vi "GetLastCharacterInformation.vi"(8 "error in (no error)":errorcluster, 10 "Right Text Information":T1, 11 "EAN-13 In":refnum<class "EAN-13.lvclass">) -> (0 "error out":errorcluster, 2 "Text Information":T1, 3 "EAN-13 out":refnum<class "EAN-13.lvclass">)   [LabVIEW 2013, in "BarCodes.lvlib" / "EAN-13.lvclass"]
uses:
  EAN-13.lvclass
  BarCode/TextPosition.ctl
  BarCodes.lvlib
  BarCode/BarCode.lvclass
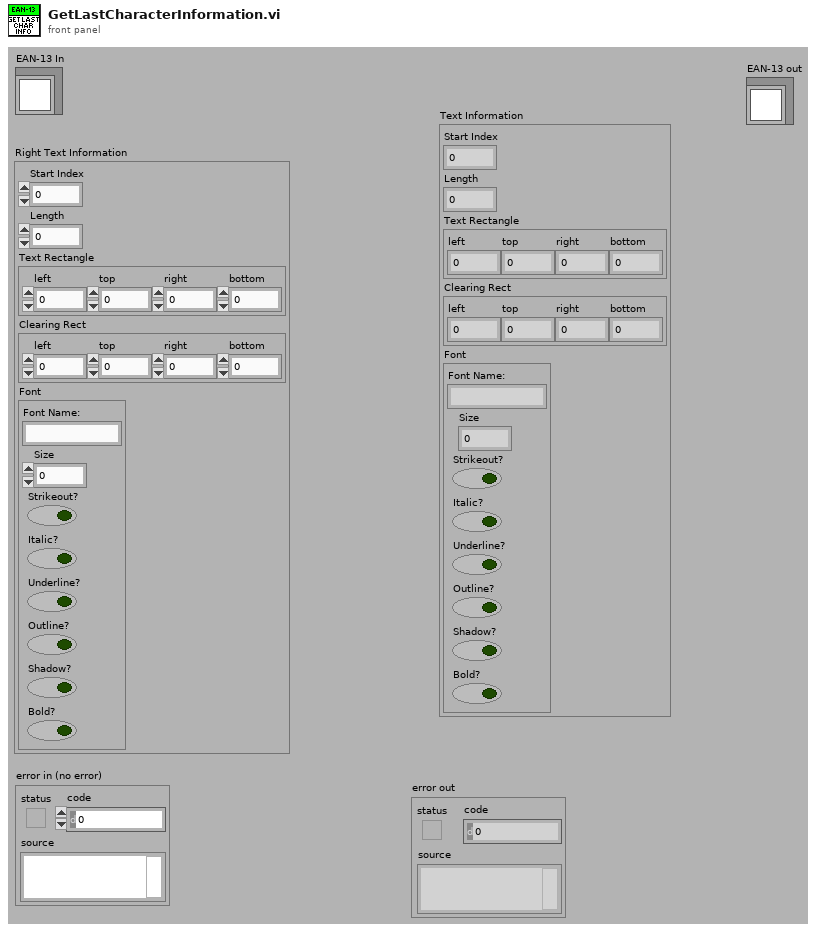
[diagram p1: front panel]
types:
  T1 = typedef "BarCodes.lvlib/BarCode.lvclass/TextPosition.ctl" = cluster{"Start Index":u8, "Length":u8, "Text Rectangle":cluster{"left":i16, "top":i16, "right":i16, "bottom":i16}, "Clearing Rect":cluster{"left":i16, "top":i16, "right":i16, "bottom":i16}, "Font":cluster{"Font Name:":string, "Size":i16, "Strikeout?":bool, "Italic?":bool, "Underline?":bool, "Outline?":bool, "Shadow?":bool, "Bold?":bool}}
  T2 = cluster{"left":i16, "top":i16, "right":i16, "bottom":i16}
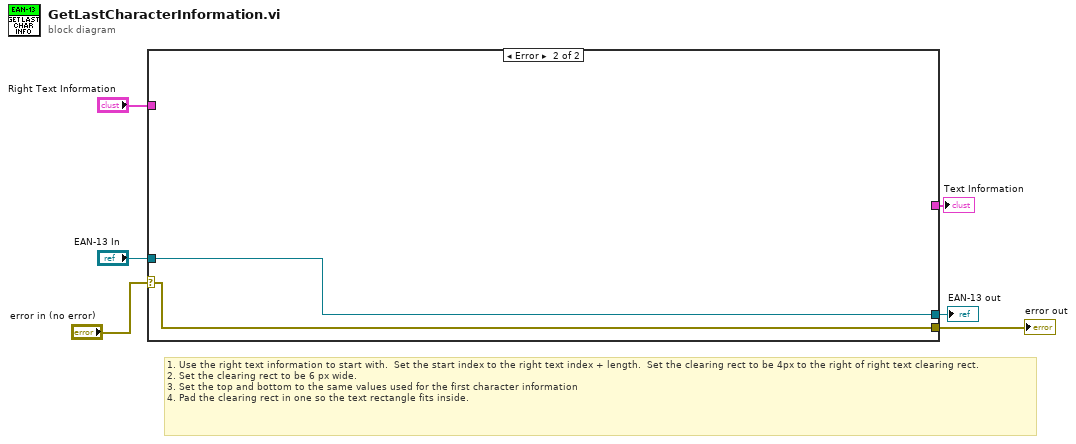
[diagram p0: block diagram]
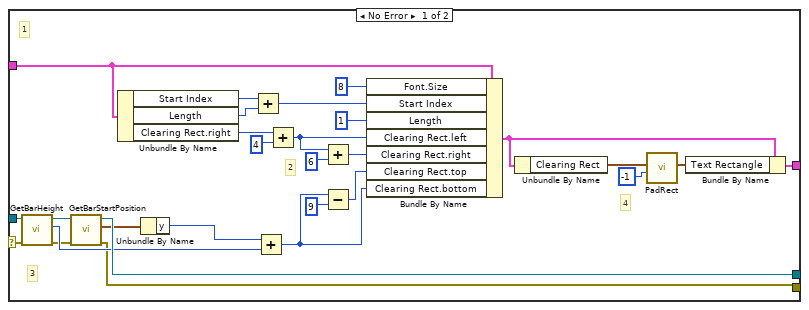
[diagram p2: hidden frame]
diagram:
  # "1. Use the right text information to start with.  Set the start index to the right text index + length.  Set the clearing rect to be 4px to the right of right text clearing rect.\n2. Set the clearing rect to be 6 px wide.\n3. Set the top and bottom to the same values used for the first character information\n4. Pad the clearing rect in one so the text rectangle fits inside."
  n1 = case shown="Error" "error in (no error)" {
    selector: "error in (no error)" -> [w9 w35]
    tunnel: "Right Text Information" -> [w32 _]
    tunnel: [w22 _] -> w5
    tunnel: "EAN-13 In" -> [w16 w36]
    tunnel: [w14 w36] -> w3
    tunnel: [w7 w35] -> w1
    frame No Error {
      # "4"
      # "3"
      # "2"
      # "1"
      n2 = call-dynamic "GetBarHeight.vi"("error in (no error)"=w9, "EAN-13 in"=w16) -> ("error out"=w8:errorcluster, "Bar Height"=w13:u8, "EAN-13 out"=w15:refnum<class "EAN-13.lvclass">)  [unwired: 7 in]
      n3 = call-dynamic "GetBarStartPosition.vi"("error in (no error)"=w8, "EAN-13 in"=w15) -> ("error out"=w7:errorcluster, "Start Position"=w12:cluster{"x":i16, "y":i16}, "EAN-13 out"=w14:refnum<class "EAN-13.lvclass">)  [unwired: 7 in]
      n4 = Unbundle By Name(w32) -> ("Start Index"=w33:u8, "Length"=w34:u8, "Clearing Rect.right"=w29:i16)
      n5 = Unbundle By Name(w12) -> ("y"=w17:i16)
      n6 = Add(x=w33, y=w34) -> (x+y=w31:u8)
      n7 = Add(x=w17, y=w13) -> (x+y=w10:i16)
      n8 = Add(x=w29, y=i16 4) -> (x+y=w20:i16)
      n9 = Add(x=w20, y=i16 6) -> (x+y=w28:i16)
      n10 = Subtract(x=w10, y=i16 9) -> (x-y=w11:i16)
      n11 = Bundle By Name(cluster=w32, "Font.Size"=i16 8, "Start Index"=w31, "Length"=u8 1, "Clearing Rect.left"=w20, "Clearing Rect.right"=w28, "Clearing Rect.top"=w11, "Clearing Rect.bottom"=w10) -> (w25:T1)
      n12 = Unbundle By Name(w25) -> ("Clearing Rect"=w27:T2)
      n13 = call "PadRect.vi"("Padding"=i8 -1, "Rectagle"=w27) -> ("Padded Rectangle"=w24:T2)  [unwired: 9 in]
      n14 = Bundle By Name(cluster=w25, "Text Rectangle"=w24) -> (w22:T1)
    }
    frame Error {
    }
  }
  "Text Information" <- w5
  "EAN-13 out" <- w3
  "error out" <- w1
